vi "Custom_Append Flattened Pixmap to Report.vi"(4 "MS Office parameters":T1, 5 "VI":refnum<vi>, 6 "caption or alt string":string, 7 "alignment (default)":T3, 8 "error in (no error)":errorcluster, 9 "image data":T2, 10 "image format (jpeg)":enum32{"PNG", "JPEG", "GIF"}(ring), 11 "report in":refnum<class "NI_report.lvclass">) -> (0 "error out":errorcluster, 1 "end out (word)":i32, 2 "start out (word)":i32, 3 "report out":refnum<class "NI_report.lvclass">)   [LabVIEW 2019]
uses:
  <vilib>/Utility/NIReport.llb/HTML Report Image Alignment.ctl
  <vilib>/Utility/NIReport.llb/NI_report.lvclass
  <vilib>/picture/picture.llb/imagedata.ctl
  <vilib>/printing/ReportDocExtensions.llb/File_types_for_reports.ctl
  <vilib>/Utility/NIReport.llb/NI_ReportGenerationCore.lvlib
panel:
  in  "Suffix":string="_frontpanel"
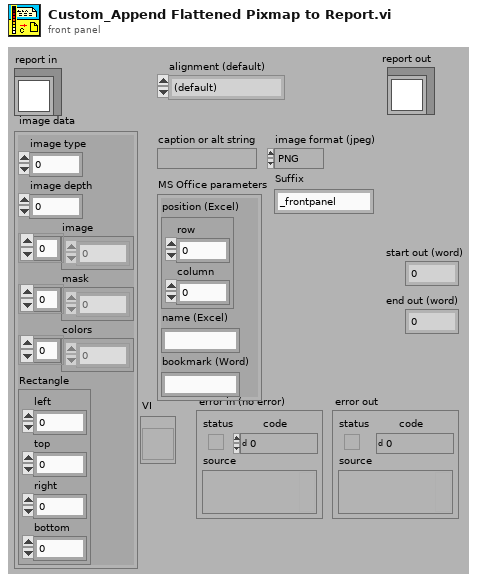
[diagram p1: front panel]
types:
  T1 = cluster{"position (Excel)":cluster{"row":i32, "column":i32}, "name (Excel)":string, "bookmark (Word)":string}
  T2 = typedef "imagedata.ctl" = cluster{"image type":i32, "image depth":i32, "image":u8[], "mask":u8[], "colors":u32[], "Rectangle":cluster{"left":i16, "top":i16, "right":i16, "bottom":i16}}
  T3 = typedef "NI_ReportGenerationCore.lvlib/HTML Report Image Alignment.ctl" = enum16{"(default)", "LEFT", "RIGHT", "TOP", "TEXTTOP", "MIDDLE", "ABSMIDDLE", "BASELINE", "BOTTOM", "ABSBOTTOM"}
  T4 = typedef "NI_ReportGenerationCore.lvlib/File_types_for_reports.ctl" = enum16{".jpg", ".png", ".html", ".gif"}
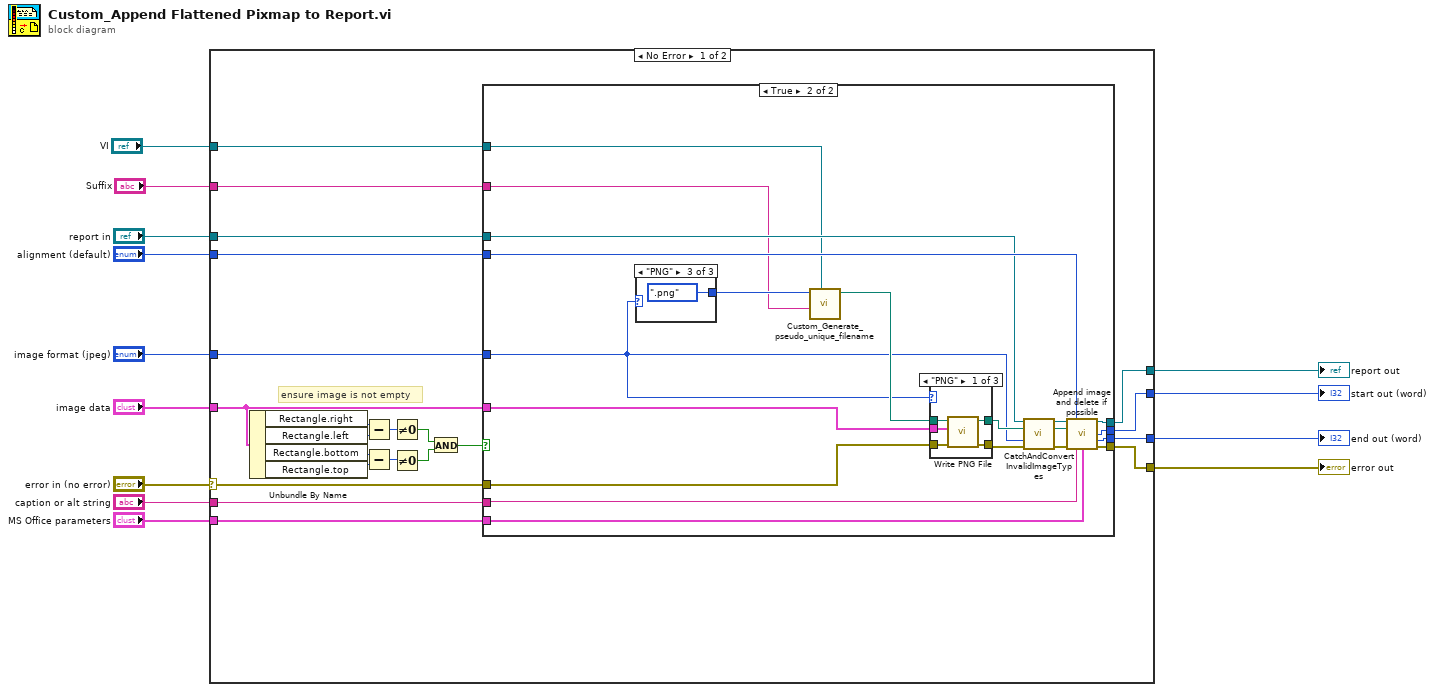
[diagram p0: block diagram]
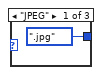
[diagram p3: hidden frame]
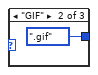
[diagram p4: hidden frame]
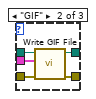
[diagram p5: hidden frame]
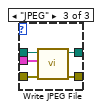
[diagram p6: hidden frame]
diagram:
  n1 = case shown="No Error" "error in (no error)" {
    selector: "error in (no error)" -> [w16 w76]
    tunnel: "caption or alt string" -> [w35 _]
    tunnel: "alignment (default)" -> [w34 _]
    tunnel: [w33 w77] -> w11
    tunnel: "report in" -> [w32 w77]
    tunnel: [w31 w76] -> w9
    tunnel: "image format (jpeg)" -> [w30 _]
    tunnel: "image data" -> [w29 _]
    tunnel: [w19 _] -> w6
    tunnel: [w18 _] -> w5
    tunnel: "MS Office parameters" -> [w17 _]
    tunnel: "VI" -> [w15 _]
    tunnel: "Suffix" -> [w14 _]
    frame No Error {
      # "ensure image is not empty"
      n2 = Unbundle By Name(w29) -> ("Rectangle.right"=w27:i16, "Rectangle.left"=w28:i16, "Rectangle.bottom"=w26:i16, "Rectangle.top"=w25:i16)
      n3 = Subtract(x=w27, y=w28) -> (x-y=w23:i16)
      n4 = Subtract(x=w26, y=w25) -> (x-y=w24:i16)
      n5 = Not Equal To 0?(x=w23) -> (x != 0?=w22:bool)
      n6 = Not Equal To 0?(x=w24) -> (x != 0?=w21:bool)
      n7 = And(x=w22, y=w21) -> (x .and. y?=w20:bool)
      n8 = case shown="True" w20 {
        tunnel: w16 -> [w36 w57]
        tunnel: w35 -> [_ w56]
        tunnel: w34 -> [_ w55]
        tunnel: [w37 w54] -> w33
        tunnel: w32 -> [w37 w52]
        tunnel: [w36 w49] -> w31
        tunnel: w30 -> [_ w44]
        tunnel: w29 -> [_ w43]
        tunnel: [_ w41] -> w19
        tunnel: [_ w40] -> w18
        tunnel: w17 -> [_ w42]
        tunnel: w15 -> [_ w39]
        tunnel: w14 -> [_ w38]
        frame False {
        }
        frame True {
          n9 = case shown="\"PNG\"" w44 {
            tunnel: [File_types_for_reports.".jpg" ("file type(.jpg)") File_types_for_reports.".gif" ("file type(.jpg)") File_types_for_reports.".png" ("file type(.jpg)")] -> w46
            frame "JPEG" {
            }
            frame "GIF" {
            }
            frame "PNG" {
            }
          }
          n10 = call "Custom_Generate_pseudo_unique_filename.vi"("VI"=w39, "Suffix"=w38, "file type(.jpg)"=w46) -> ("generated path"=w45:path)  [unwired: 6 in, 2 out]
          n11 = case shown="\"PNG\"" w44 {
            tunnel: w57 -> [w63 w70 w73]
            tunnel: [w62 w69 w71] -> w47
            tunnel: [w61 w66 w72] -> w53
            tunnel: w45 -> [w65 w68 w75]
            tunnel: w43 -> [w64 w67 w74]
            frame "PNG" {
              n12 = call <vilib>:"Write PNG File.vi"("error in (no error)"=w63, "image data"=w64, "path to PNG file"=w65) -> ("error out"=w62:errorcluster, "path"=w61:path)  [unwired: 7 in]
            }
            frame "GIF" {
              n13 = call <vilib>:"Write GIF File.vi"("error in (no error)"=w70, "image data"=w67, "path to GIF file"=w68) -> ("error out"=w69:errorcluster, "path"=w66:path)  [unwired: 7 in]
            }
            frame "JPEG" {
              n14 = call <vilib>:"Write JPEG File.vi"("error in (no error)"=w73, "image data"=w74, "path to JPEG file"=w75) -> ("error out"=w71:errorcluster, "path"=w72:path)  [unwired: 7 in]
            }
          }
          n15 = call-dynamic "CatchAndConvertInvalidImageTypes.vi"("report in"=w52, "path to image"=w53, "image format (jpeg)"=w44, "error in (no error)"=w47) -> ("report out"=w51:refnum<class "NI_report.lvclass">, "path to image out"=w50:path, "error out"=w48:errorcluster)  [unwired: 9 in]
          n16 = call-dynamic "Append image and delete if possible.vi"("report in"=w51, "alignment (default)"=w55, "path to image"=w50, "error in (no error)"=w48, "caption or alternative string"=w56, "MS Office parameters"=w42) -> ("report out"=w54:refnum<class "NI_report.lvclass">, "start out Word)"=w41:i32, "end out Word)"=w40:i32, "error out"=w49:errorcluster)  [unwired: 6 in]
        }
      }
    }
    frame Error {
    }
  }
  "report out" <- w11
  "error out" <- w9
  "start out (word)" <- w6
  "end out (word)" <- w5
